vi "EmptyPosition.vi"(0 "Chessboard in":T1, 5 "ItemIndex":T2, 11 "error in (no error)":errorcluster) -> (4 "Chessboard out":T1, 6 "ItemIndex out":T2, 8 "EmptyPosition?":bool, 15 "error out":errorcluster)   [LabVIEW 2009]
uses:
  Controls/ItemIndex.ctl
  Controls/Chess.ctl
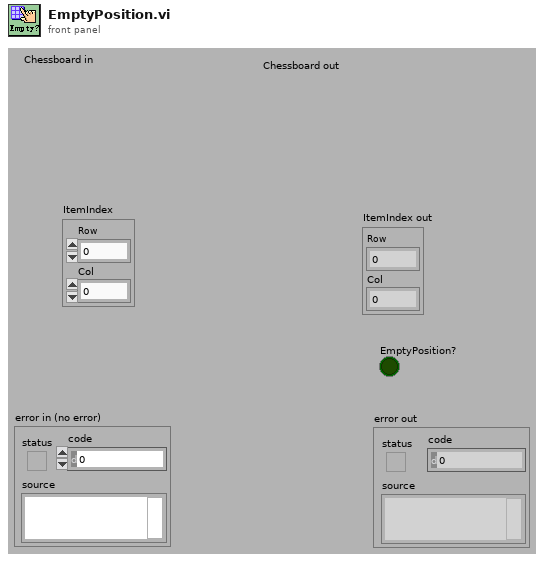
[diagram p1: front panel]
types:
  T1 = typedef "Chess.ctl" = u16[][]
  T2 = typedef "ItemIndex.ctl" = cluster{"Row":i32, "Col":i32}
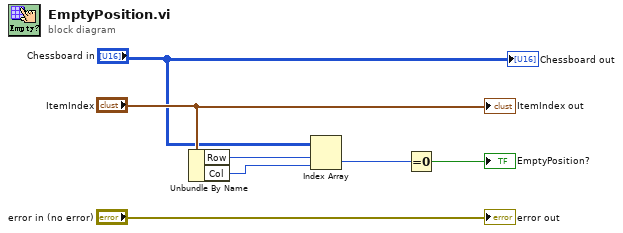
[diagram p0: block diagram]
diagram:
  n1 = Unbundle By Name("ItemIndex") -> ("Row"=w6:i32, "Col"=w5:i32)
  n2 = Index Array(array="Chessboard in", index (row)=w6, index (col)=w5) -> (element=w4:u16)
  n3 = Equal To 0?(x=w4) -> (x = 0?=→"EmptyPosition?":bool)
  "error out" <- "error in (no error)"
  "ItemIndex out" <- "ItemIndex"
  "Chessboard out" <- "Chessboard in"
